vi "5492_AutonomousStraight.vi"(9 "Length":dbl=3000.0, 10 "Position Goal":dbl, 11 "RobotDriveDevRef (Input)":T1={"DevStatus"={"status"=FALSE, "code"=0, "source"=""}, "Motors[]"=[], "Square Inputs"=FALSE, "Max Output"=1.0}) -> (3 "RobotDriveDevRef (Output)":T1={"DevStatus"={"status"=FALSE, "code"=0, "source"=""}, "Motors[]"=[], "Square Inputs"=FALSE, "Max Output"=1.0})   [LabVIEW 2017]
uses:
  <vilib>/Rock Robotics/WPI/RobotDrive/WPI_RobotDriveDevRef.ctl
  <vilib>/Rock Robotics/WPI/MotorControl/WPI_MotorControlDeviceRef.ctl
  <vilib>/Rock Robotics/WPI/MotorControl/WPI_MotorControlType.ctl
  <vilib>/Rock Robotics/SystemInterfaces/DIO/FPGA_DIOPWMChannel.ctl
  <vilib>/Rock Robotics/WPI/PWM/WPI_PWMDeadband.ctl
  <vilib>/Rock Robotics/SystemInterfaces/DIO/FPGA_DIOChannel.ctl
  5492_WPI_RobotDriveMotorSelectorEnum.ctl
  Public/Documents/Cross The Road Electronics/Phoenix-LabVIEW/Motor Controller/Controls/CTRE_Phoenix_MotorControl_ControlMode.ctl
  <vilib>/Rock Robotics/WPI/RobotDrive/WPI_RobotDriveSafetyCheck.vi
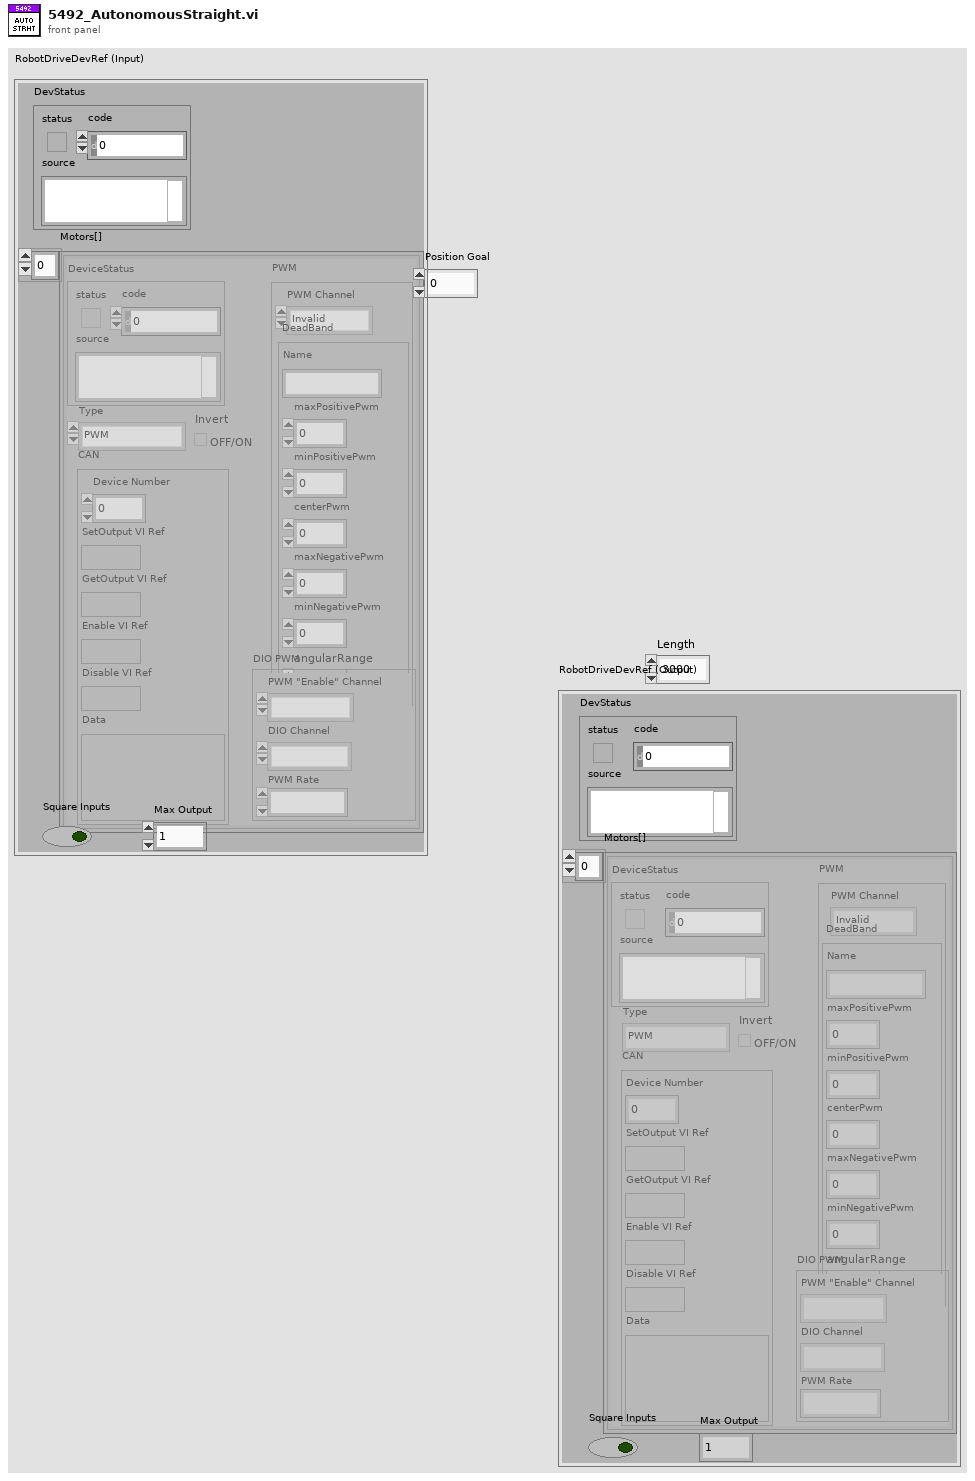
[diagram p1: front panel]
types:
  T1 = typedef "WPI_RobotDriveDevRef.ctl" = cluster{"DevStatus":errorcluster, "Motors[]":T2[], "Square Inputs":bool, "Max Output":dbl}
  T2 = typedef "WPI_MotorControlDeviceRef.ctl" = cluster{"DeviceStatus":errorcluster, "Type":T3, "PWM":cluster{"PWM Channel":T4, "DeadBand":T5}, "CAN":cluster{"Device Number":u8, "SetOutput VI Ref":variant, "GetOutput VI Ref":variant, "Enable VI Ref":variant, "Disable VI Ref":variant, "Data":variant}, "Invert":bool, "DIO PWM":cluster{"PWM \"Enable\" Channel":T4, "DIOChannel":T6, "PWM Rate":dbl}}
  T3 = typedef "WPI_MotorControlType.ctl" = enum16{"PWM", "CAN", "DIO PWM"}
  T4 = typedef "FPGA_DIOPWMChannel.ctl" = enum8{"PWM 0", "PWM 1", "PWM 2", "PWM 3", "PWM 4", "PWM 5", "PWM 6", "PWM 7", "PWM 8", "PWM 9", "PWM MXP 0", "PWM MXP 1", "PWM MXP 2", "PWM MXP 3", "PWM MXP 4", "PWM MXP 5", "PWM MXP 6", "PWM MXP 7", "PWM MXP 8", "PWM MXP 9", "Invalid"}
  T5 = typedef "WPI_PWMDeadband.ctl" = cluster{"Name":string, "maxPositivePwm":i32, "minPositivePwm":i32, "centerPwm":i32, "maxNegativePwm":i32, "minNegativePwm":i32, "angularRange":u16}
  T6 = typedef "FPGA_DIOChannel.ctl" = enum8{"DIO 0", "DIO 1", "DIO 2", "DIO 3", "DIO 4", "DIO 5", "DIO 6", "DIO 7", "DIO 8", "DIO 9", "DIO MXP 0", "DIO MXP 1", "DIO MXP 2", "DIO MXP 3", "DIO MXP 4", "DIO MXP 5", "DIO MXP 6", "DIO MXP 7", "DIO MXP 8", "DIO MXP 9", "DIO MXP 10", "DIO MXP 11", "DIO MXP 12", "DIO MXP 13", "DIO MXP 14", "DIO MXP 15", "SPI Port CS1", "SPI Port CS2", "SPI Port CS3", "SPI Port MISO", "SPI Port MOSI", "Invalid"}
  T7 = typedef "CTRE_Phoenix_MotorControl_ControlMode.ctl" = u16
  T8 = typedef "5492_WPI_RobotDriveMotorSelectorEnum.ctl" = enum16{"Front left motor", "Front right motor", "Back left motor", "Back right motor"}
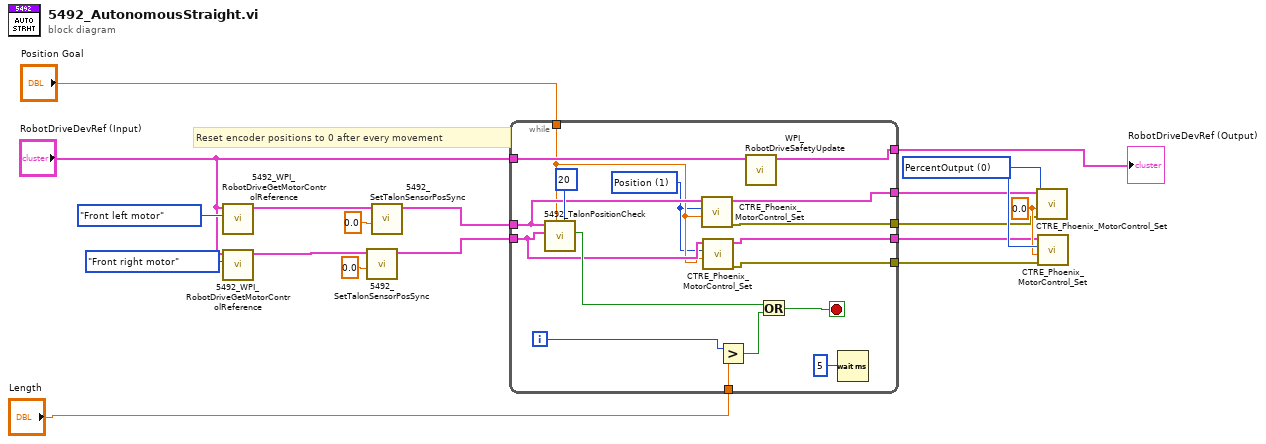
[diagram p0: block diagram]
diagram:
  w7 = T7 0 items=["PercentOutput"=0, "Position"=1, "Velocity"=2, "Current"=3, "Follower"=5, "MotionProfile"=6, "MotionMagic"=7, "MotionMagicArc"=8, "MotionProfileArc"=10, "Disabled"=15] ("Control Mode")
  w6 = 0.0 ("Output")
  # "Reset encoder positions to 0 after every movement"
  n1 = call "5492_WPI_RobotDriveGetMotorControlReference.vi"("MotorIndex"=5492_WPI_RobotDriveMotorSelectorEnum."Front left motor", "RobotDriveDevRef"="RobotDriveDevRef (Input)") -> ("MotorControlDeviceRef"=w15:T2)  [unwired: 9 out]
  n2 = call "5492_WPI_RobotDriveGetMotorControlReference.vi"("MotorIndex"=5492_WPI_RobotDriveMotorSelectorEnum."Front right motor", "RobotDriveDevRef"="RobotDriveDevRef (Input)") -> ("MotorControlDeviceRef"=w13:T2)  [unwired: 9 out]
  n3 = call "5492_SetTalonSensorPosSync.vi"("Pos"=0.0 ("New Sensor Position"), "CAN Talon SRX Ref In"=w13) -> ("CAN Talon SRX Ref Out"=w12:T2)  [unwired: 8 in, 1 out]
  n4 = call "5492_SetTalonSensorPosSync.vi"("Pos"=0.0 ("New Sensor Position"), "CAN Talon SRX Ref In"=w15) -> ("CAN Talon SRX Ref Out"=w11:T2)  [unwired: 8 in, 1 out]
  n5 = while {
    tunnel: w12 -> [w26]
    tunnel: w11 -> [w27]
    tunnel: "Length" -> [w31]
    tunnel: "Position Goal" -> [w25]
    tunnel: "RobotDriveDevRef (Input)" -> [w28]
    tunnel: [w23] -> w5
    tunnel: [w22] -> w4
    tunnel: [w21] -> w3
    tunnel: [w20] -> w2
    tunnel: [w19] -> w1
    i -> [w32]
    stop <- w35 stop-if-true
    w24 = T7 1 items=["PercentOutput"=0, "Position"=1, "Velocity"=2, "Current"=3, "Follower"=5, "MotionProfile"=6, "MotionMagic"=7, "MotionMagicArc"=8, "MotionProfileArc"=10, "Disabled"=15] ("Control Mode")
    n6 = call "5492_TalonPositionCheck.vi"("Margin of Error"=20, "Position Goal"=w25, "CAN Talon SRX Ref Right"=w26, "CAN Talon SRX Ref Left"=w27) -> ("Goal Achieved"=w34:bool)  [unwired: 7 in]
    n7 = call "CTRE_Phoenix_MotorControl_Set.vi"("Output"=w25, "Control Mode"=w24, "PhoenixMotorControlDevRef"=w27) -> ("error out"=w21:errorcluster, "PhoenixMotorControlDevRef"=w23:T2)  [unwired: 7 in]
    n8 = call "CTRE_Phoenix_MotorControl_Set.vi"("Output"=w25, "Control Mode"=w24, "PhoenixMotorControlDevRef"=w26) -> ("error out"=w20:errorcluster, "PhoenixMotorControlDevRef"=w22:T2)  [unwired: 7 in]
    n9 = Greater?(x=w32, y=w31) -> (0:w33:bool)
    n10 = call <vilib>:"WPI_RobotDriveSafetyUpdate.vi"("RobotDriveDevRef"=w28) -> ("RobotDriveDevRef"=w19:T1)  [unwired: 1 in, 9 out]
    n11 = Or(x=w34, y=w33) -> (x .or. y?=w35:bool)
    n12 = Wait (ms)(milliseconds to wait=u32 5) -> ()  [unwired: 1 out]
  }
  "RobotDriveDevRef (Output)" <- w1
  n13 = call "CTRE_Phoenix_MotorControl_Set.vi"("error in (no error)"=w3, "Output"=w6, "Control Mode"=w7, "PhoenixMotorControlDevRef"=w5) -> ()  [unwired: 6 in, 2 out]
  n14 = call "CTRE_Phoenix_MotorControl_Set.vi"("error in (no error)"=w2, "Output"=w6, "Control Mode"=w7, "PhoenixMotorControlDevRef"=w4) -> ()  [unwired: 6 in, 2 out]
